vi "Read TopRef.vi"(8 "error in (no error)":errorcluster, 11 "UIActorTop2 in":refnum<class "MouseHandle.lvclass">) -> (0 "error out":errorcluster, 2 "TopRef":T1, 3 "UIActorTop2 out":refnum<class "MouseHandle.lvclass">)   [LabVIEW 2021, in "MouseHandle.lvlib" / "MouseHandle.lvclass"]
uses:
  MouseHandle.lvclass
  TopRef.ctl
  MouseHandle.lvclass/MouseHandle.ctl
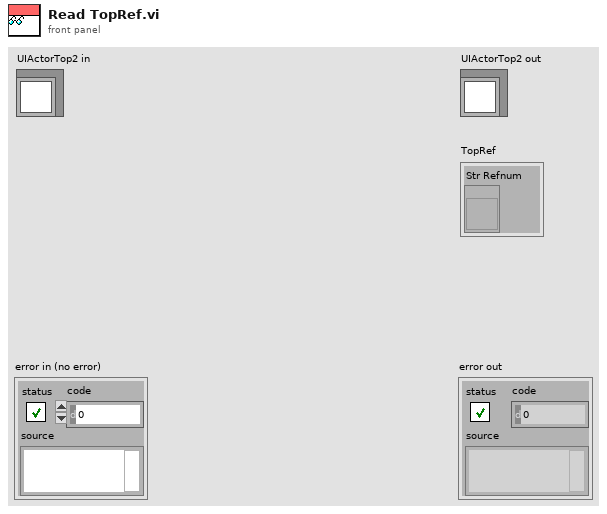
[diagram p1: front panel]
types:
  T1 = typedef "MouseHandle.lvlib/MouseHandle.lvclass/TopRef.ctl" = cluster{"Str Refnum":refnum<vi>}
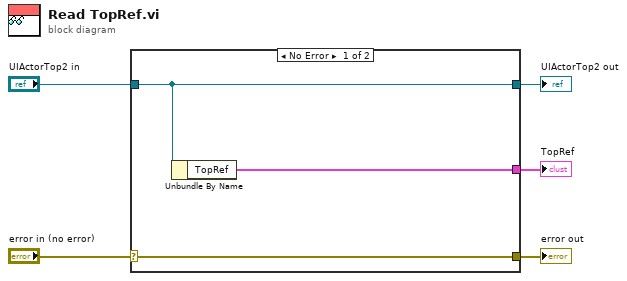
[diagram p0: block diagram]
diagram:
  n1 = case shown="No Error" "error in (no error)" {
    selector: "error in (no error)" -> [w8 w9]
    tunnel: [w8 w9] -> w4
    tunnel: [w7 w10] -> w2
    tunnel: "UIActorTop2 in" -> [w7 w10]
    tunnel: [w6 _] -> w1
    frame No Error {
      n2 = Unbundle By Name(w7) -> ("TopRef"=w6:T1)
    }
    frame Error {
    }
  }
  "error out" <- w4
  "UIActorTop2 out" <- w2
  "TopRef" <- w1
